vi "Read Output Till Settle.vi"(7 "timeout [ms]":u32, 8 "error in":errorcluster, 10 "settled for [ms]":u32, 11 "pipe in":T1) -> (0 "error out":errorcluster, 2 "read buffer":string, 3 "pipe out":T1, 5 "bytes remaining":i32)   [LabVIEW 2013, in "GOLPI library.lvlib"]
doc: "Continually reads output of GNU Octave. If no new data appears in the buffer for at least 'settled for' miliseconds, reading stops. If timeout is exceeded, returns only part of buffer and returns number of bytes remaining in the stdout buffer."
uses:
  GOLPI library.lvlib
  LV Process.lvlibp/Pipe Handle.ctl
  LV Process.lvlibp
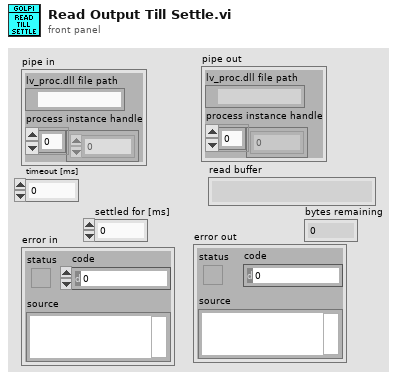
[diagram p1: front panel]
types:
  T1 = typedef "LV Process.lvlibp/Pipe Handle.ctl" = cluster{"lv_proc.dll file path":path, "process instance handle":u32[]}
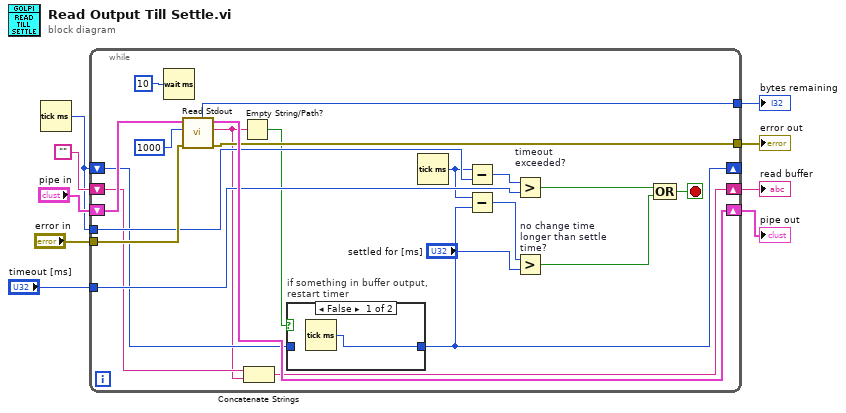
[diagram p0: block diagram]
diagram:
  n1 = Tick Count (ms)() -> (millisecond timer value=w1:u32)
  n2 = while {
    tunnel: [w29] -> w7
    tunnel: "error in" -> [w28]
    tunnel: [w23] -> w4
    shift-right: [w30] -> w8
    shift-left: "pipe in" -> [w31]
    shift-right: [w27] -> w5
    shift-left: "" -> [w18]
    tunnel: w1 -> [w26]
    tunnel: "timeout [ms]" -> [w24]
    shift-right: [w12] -> _
    shift-left: w1 -> [w17]
    stop <- w21 stop-if-true
    n3 = Wait (ms)(milliseconds to wait=u32 10) -> ()  [unwired: 1 out]
    n4 = call "Read Stdout.vi"("error in"=w28, "byte count"=1000, "pipe in"=w31) -> ("error out"=w29:errorcluster, "read buffer"=w13:string, "pipe out"=w30:T1, "bytes remaining"=w23:i32)  [unwired: 3 in, 2 out]
    n5 = Empty String/Path?(string/path=w13) -> (empty?=w14:bool)
    n6 = Concatenate Strings(w18, w13) -> (w27:string)
    n7 = case "if something in buffer output,\nrestart timer" shown="False" w14 {
      tunnel: [w32 w33] -> w12
      tunnel: w17 -> [_ w33]
      frame False {
        n8 = Tick Count (ms)() -> (millisecond timer value=w32:u32)
      }
      frame True {
      }
    }
    n9 = Tick Count (ms)() -> (millisecond timer value=w10:u32)
    n10 = Subtract(x=w10, y=w26) -> (x-y=w25:u32)
    n11 = Subtract(x=w10, y=w12) -> (x-y=w11:u32)
    n12 = Greater? "timeout\nexceeded?"(x=w25, y=w24) -> (0:w22:bool)
    n13 = Greater? "no change time\nlonger than settle\ntime?"(x=w11, y="settled for [ms]") -> (0:w15:bool)
    n14 = Compound Arithmetic op=OR(w22, w15) -> (w21:bool)
  }
  "pipe out" <- w8
  "error out" <- w7
  "read buffer" <- w5
  "bytes remaining" <- w4
